vi "Execution Control Global.vi"() -> ()   [LabVIEW 2013]
panel:
  out "Stop":bool
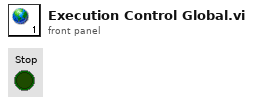
[diagram p1: front panel]
diagram:
